vi "温度上传.vi"(2 "温度最低限定值":dbl, 3 "温度最高限定值":dbl, 4 "当前温度":dbl) -> (0 "报警灯":bool, 1 "温度曲线":T1(graph))   [LabVIEW 2013]
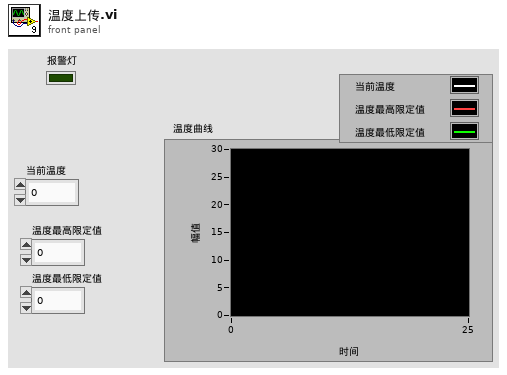
[diagram p1: front panel]
types:
  T1 = cluster{"当前温度":dbl, "温度最高限定值":dbl, "温度最低限定值":dbl}
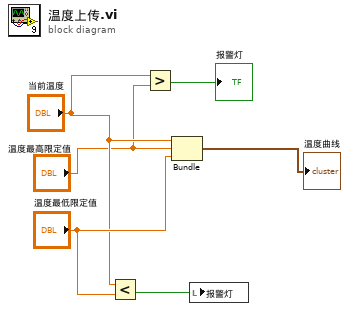
[diagram p0: block diagram]
diagram:
  n1 = Less?(x="当前温度", y="温度最低限定值") -> (x < y?=w6:bool)
  n2 = Greater?(x="当前温度", y="温度最高限定值") -> (0:→"报警灯":bool)
  n3 = Bundle("当前温度"="当前温度", "温度最高限定值"="温度最高限定值", "温度最低限定值"="温度最低限定值") -> (→"温度曲线":T1)  [unwired: 1 in]
  n4 = local write "报警灯"(w6) -> ()
